vi "Init(Update ref).vi"(8 "error in (no error)":errorcluster, 10 "Interface Cluster":T1, 11 "Domino Laser module Class in":refnum<class "Domino Laser module Class.lvclass">) -> (0 "error out":errorcluster, 3 "Domino Laser module Class out":refnum<class "Domino Laser module Class.lvclass">)   [LabVIEW 2015, in "Domino LM.lvlib" / "Domino Laser module Class.lvclass"]
uses:
  CTRLS/Domino Laser module Class.lvclass
  CTRLS/Printer interface cluster.ctl
  ARCH/Message Queue/Message Cluster.ctl
  CTRLS/Open Batch Data.ctl
  CTRLS/Printer Message settings.ctl
  CTRLS/Domino Laser module Class.lvclass/Domino Laser module Class.ctl
  ARCH/Message Queue/Message Queue.lvlib
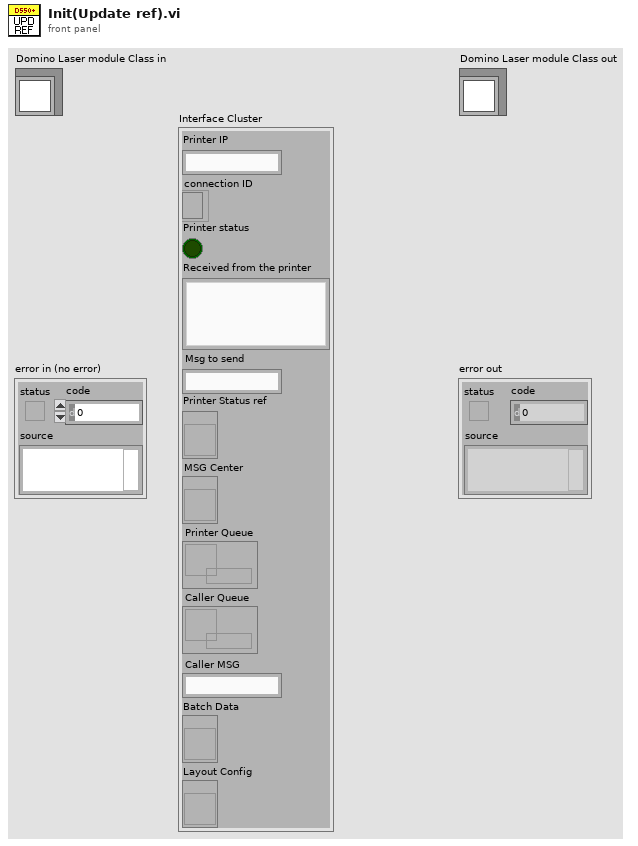
[diagram p1: front panel]
types:
  T1 = typedef "Printer interface cluster.ctl" = cluster{"Printer IP":string, "connection ID":refnum<k5>, "Printer status":bool, "Received from the printer":string, "Msg to send":string, "Printer Status ref":refnum<vi>, "MSG Center":refnum<vi>, "Printer Queue":refnum<queue>, "Caller Queue":refnum<queue>, "Caller MSG":string, "Batch Data":refnum<vi>, "Layout Config":refnum<vi>}
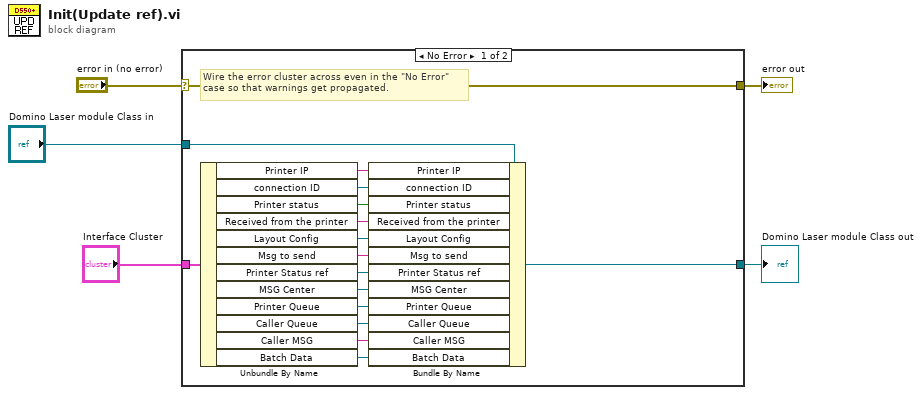
[diagram p0: block diagram]
diagram:
  n1 = case shown="No Error" "error in (no error)" {
    selector: "error in (no error)" -> [w21 w23]
    tunnel: [w21 w23] -> w4
    tunnel: [w19 w22] -> w2
    tunnel: "Domino Laser module Class in" -> [w20 w22]
    tunnel: "Interface Cluster" -> [w18 _]
    frame No Error {
      # "Wire the error cluster across even in the \"No Error\"\ncase so that warnings get propagated."
      n2 = Unbundle By Name(w18) -> ("Printer IP"=w17:string, "connection ID"=w16:refnum<k5>, "Printer status"=w15:bool, "Received from the printer"=w14:string, "Layout Config"=w13:refnum<vi>, "Msg to send"=w12:string, "Printer Status ref"=w11:refnum<vi>, "MSG Center"=w10:refnum<vi>, "Printer Queue"=w9:refnum<queue>, "Caller Queue"=w8:refnum<queue>, "Caller MSG"=w7:string, "Batch Data"=w6:refnum<vi>)
      n3 = Bundle By Name(cluster=w20, "Printer IP"=w17, "connection ID"=w16, "Printer status"=w15, "Received from the printer"=w14, "Layout Config"=w13, "Msg to send"=w12, "Printer Status ref"=w11, "MSG Center"=w10, "Printer Queue"=w9, "Caller Queue"=w8, "Caller MSG"=w7, "Batch Data"=w6) -> (w19:refnum<class "Domino Laser module Class.lvclass">)
    }
    frame Error {
    }
  }
  "error out" <- w4
  "Domino Laser module Class out" <- w2
